vi "Receiver_Chirp_PG_DEMO.vi"() -> ()   [LabVIEW 2017]
uses:
  <vilib>/DAQmx/read.llb/DAQmx Read (Analog Wfm 1Chan NSamp).vi
  <vilib>/DAQmx/create/channels.llb/DAQmx Create Channel (AI-Voltage-Basic).vi
  <vilib>/DAQmx/configure/timing.llb/DAQmx Timing (Sample Clock).vi
  <vilib>/DAQmx/miscellaneous.llb/DAQmx Fill In Error Info.vi
  <vilib>/Analysis/3filter.llb/FIR Filter (DBL).vi
  <vilib>/Analysis/NI_AALBase.lvlib
panel:
  out "Dechirp. level(dB)":dbl
  out "Rx. level(dB)":dbl
  in  "Range(m)":dbl=10.0 format="%#_6p"
  in  "Ref.":bool
  in  "Rx.Gain(dB)":dbl=32.0 format="%#_6p"
  in  "Tx.V(Vpp)":dbl=24.0 format="%#_6p"
  in  "RVS(dB)":dbl=-197.0 format="%#_6p"
  in  "TVR(dB)":dbl=133.0 format="%#_6p"
  out "Count":i32
  out "숫자형 인디케이터 2":dbl
  out ",,":dbl[](array[numeric])
  in  "재생 버튼":bool
  out "Save":i32(slide) scale=0.0..40.0
  out "Acqusition":i32(slide) scale=0.0..40.0
  out "Dechirp":waveform(dbl)(graph)
  out "Acquired Data 2":waveform(dbl)(graph)={"t0"=timestamp(0 s since 1904-01-01), "dt"=5e-06, "Y"=[]}
  in  "End Freq. (Hz)":dbl=34000.0 format="%#_6p"
  in  "Freq. (Hz)":dbl=30000.0 format="%#_6p"
  in  "Pulse Length(sec)":dbl=0.004 format="%#_6p"
  in  "Read (sec)":i32=2 format="%.0p"
  in  "#S":i32=10000 format="%.0p"
  in  "Fs":dbl=200000.0 format="%#_6p"
  in  "Channel":tag="Dev1/ai0"
  in  "Device":tag="Dev1"
  out "Acquired Data":waveform(dbl)(graph)={"t0"=timestamp(3635219585.299205 s since 1904-01-01), "dt"=4.999999999999959e-06, "Y"=[], "attributes"=variant("NI_ChannelName"=variant(string "Dev1/ai0"), "NI_UnitDescription"=variant(string "Volts"))}
  in  "File Path":path=path "C:/Users/FishingNetID/Desktop/Source code/이기배/E-어구/오이도해상시험/RawData/4ms_Upchirp_10m_"
  # "Processing Gain(PG) Measurment"
  # "Device"
  # "Parameter"
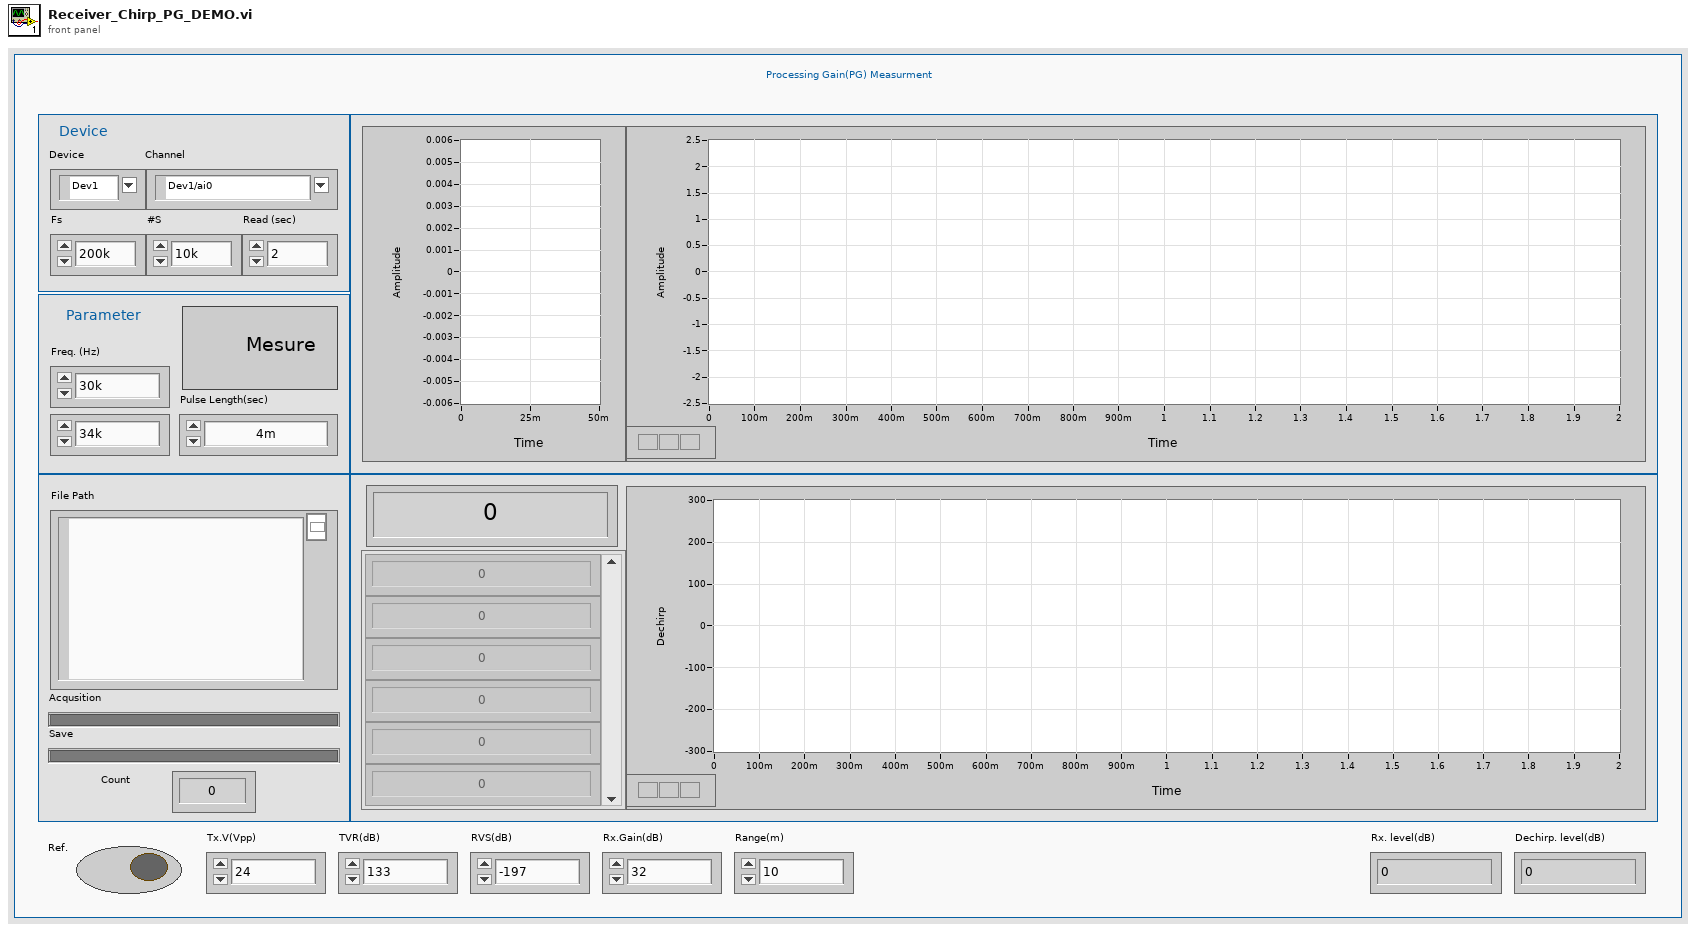
[diagram p1: front panel]
types:
  T1 = enum16{"open", "open or create", "create or replace", "create", "open (read-only)"}
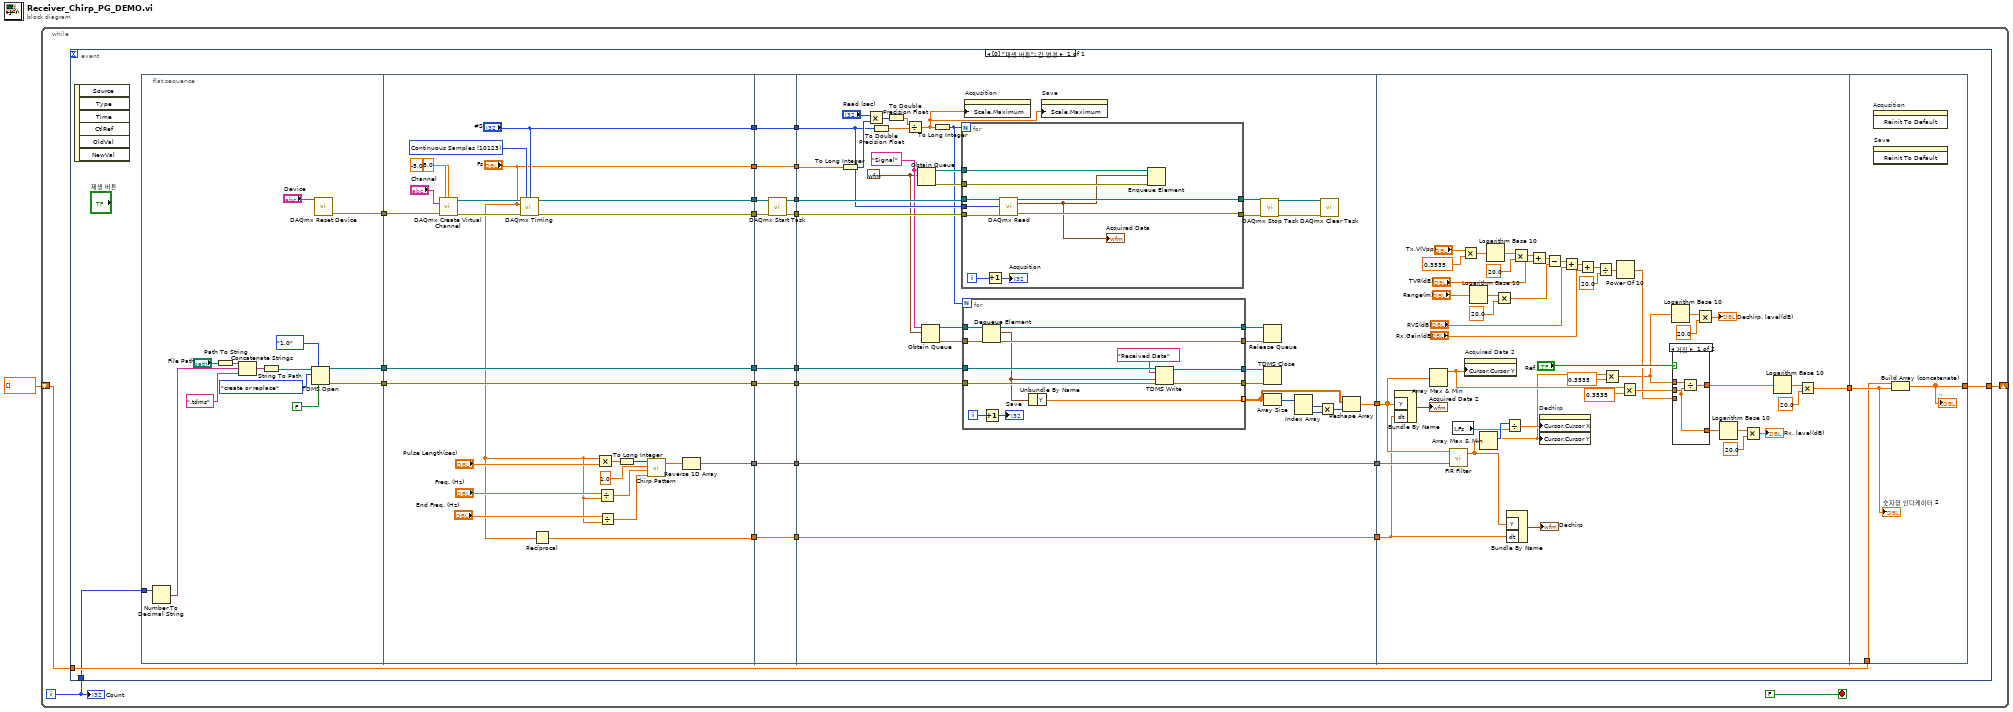
[diagram p0: block diagram]
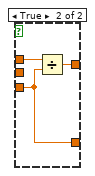
[diagram p2: hidden frame]
diagram:
  n1 = while {
    shift-right: [w4] -> _
    shift-left: dbl[] [] -> [w3]
    i -> [w2]
    stop <- FALSE stop-if-true
    n2 = event shown="[0] \"재생 버튼\": 값 변경" {
      selector: _ -> [_]
      dyn-events: _ -> [_]
      timeout: _ -> [_]
      tunnel: [w8] -> w4
      tunnel: w3 -> [w7]
      tunnel: w2 -> [w6]
      event "재생 버튼": Value Change {
        n3 = event-data() -> ()  [unwired: 1 in, 6 out]
        n4 = flat-sequence {
          tunnel: [w44] -> w31
          tunnel: [w43] -> w30
          tunnel: [w42] -> w29
          tunnel: w6 -> [w33]
          tunnel: w31 -> [w69]
          tunnel: [w64] -> w28
          tunnel: [w63] -> w27
          tunnel: ["#S"] -> w26
          tunnel: ["Fs"] -> w25
          tunnel: [w58] -> w24
          tunnel: [w59] -> w23
          tunnel: w30 -> [w59]
          tunnel: w29 -> [w58]
          tunnel: [w54] -> w22
          tunnel: [w52] -> w21
          tunnel: w28 -> [w78]
          tunnel: w27 -> [w79]
          tunnel: [w77] -> w18
          tunnel: [w76] -> w17
          tunnel: [w75] -> w16
          tunnel: w26 -> [w75]
          tunnel: [w74] -> w15
          tunnel: w25 -> [w74]
          tunnel: [w73] -> w19
          tunnel: w24 -> [w73]
          tunnel: [w72] -> w20
          tunnel: w23 -> [w72]
          tunnel: [w71] -> w14
          tunnel: w22 -> [w71]
          tunnel: [w70] -> w13
          tunnel: w21 -> [w70]
          tunnel: w20 -> [w100]
          tunnel: w19 -> [w101]
          tunnel: w18 -> [w114]
          tunnel: w17 -> [w113]
          tunnel: w16 -> [w105]
          tunnel: w15 -> [w107]
          tunnel: w14 -> [w81]
          tunnel: [w86] -> w12
          tunnel: w13 -> [w82]
          tunnel: [w82] -> w11
          tunnel: [w81] -> w10
          tunnel: w12 -> [w183]
          tunnel: w11 -> [w175]
          tunnel: w10 -> [w179]
          tunnel: [w178] -> w9
          tunnel: w9 -> [w193]
          tunnel: [w191] -> w8
          tunnel: w7 -> [w192]
          frame #0 {
            n5 = Number To Decimal String(number=w33) -> (decimal integer string=w32:string)  [unwired: 1 in]
            n6 = Path To String(path="File Path") -> (string=w37:string)
            n7 = Concatenate Strings(w37, w32, ".tdms") -> (w36:string)
            n8 = String To Path(string=w36) -> (path=w35:path)
            n9 = TDMS Open(6:FALSE ("disable buffering? (T)"), 7:enum16{"1.0", "2.0"}."1.0" ("file format version (2.0)"), 10:T1."create or replace" ("operation (0:open)"), 11:w35) -> (0:w43:errorcluster, 3:w42:refnum<k34>)  [unwired: 3 in]
            n10 = call <vilib>:"DAQmx Reset Device.vi"("device in"="Device") -> ("error out"=w44:errorcluster)  [unwired: 1 in, 13 out]
          }
          frame #1 {
            w61 = 10123 items=["Finite Samples"=10178, "Continuous Samples"=10123, "Hardware Timed Single Point"=12522] ("sample mode")
            n11 = call-poly <vilib>:"DAQmx Create Virtual Channel.vi"("maximum value"=5.0, "minimum value"=-5.0, "physical channels"="Channel", "error in"=w69) -> ("task out"=w66:refnum<k21>, "error out"=w65:errorcluster)  [unwired: 5 in, 5 out]
            n12 = call-poly <vilib>:"DAQmx Timing.vi"("task/channels in"=w66, "sample mode"=w61, "samples per channel"="#S", "rate"="Fs", "error in"=w65) -> ("task out"=w64:refnum<k21>, "error out"=w63:errorcluster)  [unwired: 2 in, 7 out]
            n13 = Reciprocal(x="Fs") -> (1/x=w52:dbl)
            n14 = Multiply(x="Fs", y="Pulse Length(sec)") -> (x*y=w51:dbl)
            n15 = Divide(x="Freq. (Hz)", y="Fs") -> (x/y=w46:dbl)
            n16 = Divide(x="End Freq. (Hz)", y="Fs") -> (x/y=w47:dbl)
            n17 = To Long Integer(number=w51) -> (32bit integer=w50:i32)
            n18 = call <vilib>:"Chirp Pattern.vi"("f2"=w47, "f1"=w46, "amplitude"=1.0, "samples"=w50) -> ("Chirp Pattern"=w49:dbl[])  [unwired: 1 out]
            n19 = Reverse 1D Array(array=w49) -> (reversed array=w54:dbl[])
          }
          frame #2 {
            n20 = call <vilib>:"DAQmx Start Task.vi"("task/channels in"=w78, "error in"=w79) -> ("task out"=w77:refnum<k21>, "error out"=w76:errorcluster)  [unwired: 12 out]
          }
          frame #3 {
            w84 = "Signal" ("이름(이름없음)")
            w83 = waveform(dbl) {"t0"=timestamp(0 s since 1904-01-01), "dt"=1.0, "Y"=[]} ("Waveform")
            n21 = To Long Integer(number=w107) -> (32bit integer=w106:i32)
            n22 = Multiply(x="Read (sec)", y=w106) -> (x*y=w103:i32)
            n23 = To Double Precision Float(number=w105) -> (double precision float=w104:dbl)
            n24 = To Double Precision Float(number=w103) -> (double precision float=w102:dbl)
            n25 = Divide(x=w102, y=w104) -> (x/y=w80:dbl)
            n26 = Obtain Queue(name (unnamed)=w84, element data type=w83) -> (queue out=w97:refnum<queue>, error out=w96:errorcluster)  [unwired: 3 in, 1 out]
            n27 = Obtain Queue(name (unnamed)=w84, element data type=w83) -> (queue out=w95:refnum<queue>, error out=w94:errorcluster)  [unwired: 3 in, 1 out]
            n28 = To Long Integer(number=w80) -> (32bit integer=w85:i32)
            n29 = for {
              N: w85 -> [_]
              tunnel: w105 -> [w133]
              tunnel: w114 -> [w137]
              tunnel: [w135] -> w112
              tunnel: w113 -> [w136]
              tunnel: [w134] -> w111
              tunnel: w97 -> [w132]
              tunnel: w96 -> [w131]
              i -> [w128]
              n30 = Increment(x=w128) -> (x+1=→"Acqusition":i32)
              n31 = call-poly <vilib>:"DAQmx Read.vi"("task/channels in"=w137, "number of samples per channel"=w133, "error in"=w136) -> ("task out"=w135:refnum<k21>, "data"=w130:waveform(dbl), "error out"=w134:errorcluster)  [unwired: 10 out]
              "Acquired Data" <- w130
              n32 = Enqueue Element(queue=w132, element=w130, error in (no error)=w131) -> ()  [unwired: 1 in, 3 out]
            }
            n33 = for {
              N: w85 -> [_]
              tunnel: w101 -> [w127]
              tunnel: [w125] -> w99
              tunnel: w100 -> [w126]
              tunnel: [w124] -> w98
              tunnel: w95 -> [w122]
              tunnel: w94 -> [w121]
              tunnel: [w120] -> w93
              tunnel: [w119] -> w92
              tunnel: [w117] -> w87 mode=indexing
              i -> [w116]
              n34 = Dequeue Element(queue=w122, error in (no error)=w121) -> (queue out=w120:refnum<queue>, element=w118:waveform(dbl), error out=w119:errorcluster)  [unwired: 2 out]
              n35 = Increment(x=w116) -> (x+1=→"Save":i32)
              n36 = Unbundle By Name(w118) -> ("Y"=w117:dbl[])
              n37 = TDMS Write(0:w127, 5:"Received Data" ("그룹 이름 입력(제목없음)"), 9:w118, 11:w126) -> (4:w125:refnum<k34>, 15:w124:errorcluster)  [unwired: 2 in, 2 out]
            }
            n38 = property on="Acqusition" class="Slide (엄격한)"("Scale.Maximum"=w80) -> ()  [unwired: 2 in, 2 out]
            n39 = property on="Save" class="Slide (엄격한)"("Scale.Maximum"=w80) -> ()  [unwired: 2 in, 2 out]
            n40 = call <vilib>:"DAQmx Stop Task.vi"("task/channels in"=w112, "error in"=w111) -> ("task out"=w110:refnum<k21>, "error out"=w109:errorcluster)  [unwired: 12 out]
            n41 = TDMS Close(8:w98, 11:w99) -> ()  [unwired: 2 out]
            n42 = Array Size(array=w87) -> (size(s)=w91:i32[])
            n43 = Release Queue(queue=w93, error in (no error)=w92) -> ()  [unwired: 4 out]
            n44 = Index Array(array=w91) -> (element #1=w89:i32, element #2=w90:i32)  [unwired: 2 in]
            n45 = Multiply(x=w89, y=w90) -> (x*y=w88:i32)
            n46 = call <vilib>:"DAQmx Clear Task.vi"("task in"=w110, "error in"=w109) -> ()  [unwired: 14 out]
            n47 = Reshape Array(w87, w88) -> (w86:dbl[])
          }
          frame #4 {
            n48 = Bundle By Name("Y"=w183, "dt"=w175) -> (→"Acquired Data 2":waveform(dbl))  [unwired: 1 in]
            n49 = Array Max & Min(array=w183) -> (max value=w149:dbl)  [unwired: 3 out]
            n50 = call-poly <vilib>:"FIR Filter.vi"("FIR Coefficients"=w179, "X"=w183) -> ("Filtered X"=w177:dbl[])  [unwired: 2 in, 1 out]
            n51 = local read "Fs"() -> (w173:dbl)
            n52 = Multiply(x="Tx.V(Vpp)", y=0.3535) -> (x*y=w169:dbl)
            n53 = property on="Acquired Data 2" class="WFGraph (엄격한)"("Cursor.Cursor Y"=w149) -> ()  [unwired: 2 in, 2 out]
            n54 = Logarithm Base 10(1:"Range(m)") -> (0:w161:dbl)
            n55 = Array Max & Min(array=w177) -> (max value=w145:dbl, max index (indices)=w174:i32)  [unwired: 2 out]
            n56 = Logarithm Base 10(1:w169) -> (0:w168:dbl)
            n57 = Multiply(x=w161, y=20.0) -> (x*y=w157:dbl)
            n58 = Divide(x=w174, y=w173) -> (x/y=w172:dbl)
            n59 = Bundle By Name("Y"=w177, "dt"=w175) -> (→"Dechirp":waveform(dbl))  [unwired: 1 in]
            n60 = Multiply(x=w168, y=20.0) -> (x*y=w166:dbl)
            n61 = Add(x=w166, y="TVR(dB)") -> (x+y=w158:dbl)
            n62 = property on="Dechirp" class="WFGraph (엄격한)"("Cursor.Cursor X"=w172, "Cursor.Cursor Y"=w145) -> ()  [unwired: 2 in, 2 out]
            n63 = Subtract(x=w158, y=w157) -> (x-y=w155:dbl)
            n64 = Add(x=w155, y="RVS(dB)") -> (x+y=w163:dbl)
            n65 = Add(x=w163, y="Rx.Gain(dB)") -> (x+y=w154:dbl)
            n66 = Divide(x=w154, y=20.0) -> (x/y=w152:dbl)
            n67 = Multiply(x=w145, y=0.3535) -> (x*y=w139:dbl)
            n68 = Power Of 10(x=w152) -> (10^x=w144:dbl)
            n69 = Multiply(x=w149, y=0.3535) -> (x*y=w147:dbl)
            n70 = Logarithm Base 10(1:w139) -> (0:w140:dbl)
            n71 = case shown="거짓" "Ref." {
              tunnel: w147 -> [w185 _]
              tunnel: [w186 w190] -> w181
              tunnel: w139 -> [w187 w189]
              tunnel: [w185 w188] -> w143
              tunnel: w144 -> [_ w188]
              frame False {
                n72 = Divide(x=w187, y=w185) -> (x/y=w186:dbl)
              }
              frame True {
                n73 = Divide(x=w189, y=w188) -> (x/y=w190:dbl)
              }
            }
            n74 = Multiply(x=w140, y=20.0) -> (x*y=→"Dechirp. level(dB)":dbl)
            n75 = Logarithm Base 10(1:w143) -> (0:w150:dbl)
            n76 = Multiply(x=w150, y=20.0) -> (x*y=→"Rx. level(dB)":dbl)
            n77 = Logarithm Base 10(1:w181) -> (0:w180:dbl)
            n78 = Multiply(x=w180, y=20.0) -> (x*y=w178:dbl)
          }
          frame #5 {
            n79 = invoke on="Acqusition" class="Slide (엄격한)" method="Reinit To Default"() -> ()  [unwired: 3 in, 3 out]
            n80 = invoke on="Save" class="Slide (엄격한)" method="Reinit To Default"() -> ()  [unwired: 3 in, 3 out]
            n81 = Build Array (concatenate)(w192, w193) -> (w191:dbl[])
            ",," <- w191
            "숫자형 인디케이터 2" <- w193
          }
        }
      }
    }
    "Count" <- w2
  }
